vi "Is Null.vi"(11 "Texture in":refnum<class "Texture.lvclass">) -> (3 "Is Null":bool)   [LabVIEW 2015, in "Texture.lvclass"]
uses:
  Texture.lvclass
  Texture.lvclass/Texture.ctl
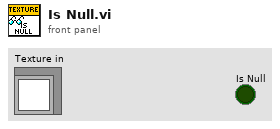
[diagram p1: front panel]
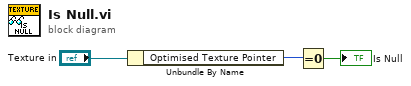
[diagram p0: block diagram]
diagram:
  n1 = Unbundle By Name("Texture in") -> ("Optimised Texture Pointer"=w2:u32)
  n2 = Equal To 0?(x=w2) -> (x = 0?=→"Is Null":bool)
